vi "ProdaNG.TestValue.Set.vi"(8 "error in (no error)":errorcluster, 9 "ReleaseId":T1, 10 "TestValue":T2 {"minimum" format="%#.3f"; "maximum" format="%#.3f"}, 11 "dbHandleIn":i32) -> (0 "error out":errorcluster, 2 "TestValue out":T2 {"minimum" format="%#.3f"; "maximum" format="%#.3f"}, 3 "dbHandle":i32)   [LabVIEW 2016]
doc: "This function returns a product structure for a product, which is identified by a part and a serial number.\nImportant information: The field 'individual' was taken over from the field 'allgemein' of the legacy data directly. Because of this most products have the value 0 further on and only a few the value 1. \nParameter:\nhandle is an Integer, which is returned by the function Login() at the creation of a new connection.\nwabcoPartId is the Id of the part.\nserialNumber is the serial number of the product for the part above.\nproduct is a pointer on a product structure, which is filled if the returncode is 0. The structure must be defined in the calling program.\n\nReturncodes:\n0 No error\n< 0 ORACLE Error code\n6 (ERROR_INVALID_HANDLE) in case of an invalid handle\n1403 Record does not exist"
uses:
  Controls/ProdaNG.TestValue.ctl
  Controls/ProdaNG.ReleaseId.ctl
  Controls/ProdaNG.TestValueSize.ctl
  prodllNG.dll
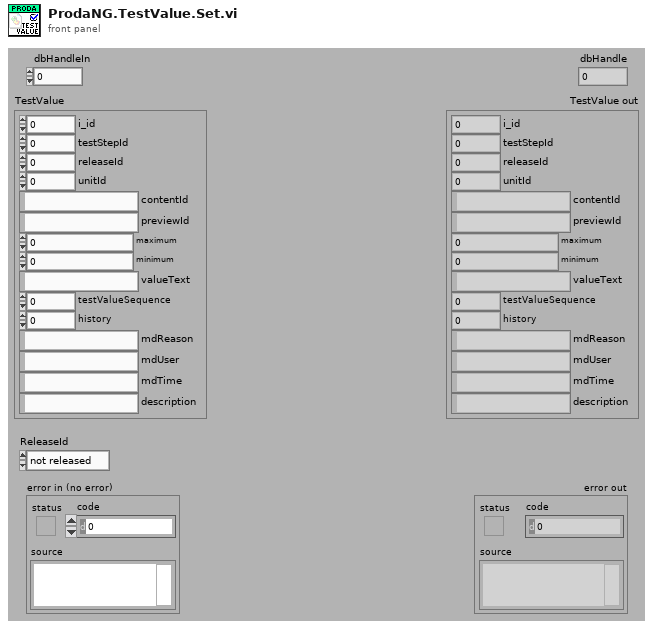
[diagram p1: front panel]
types:
  T1 = typedef "ProdaNG.ReleaseId.ctl" = enum16{"not released", "released", "was released"}
  T2 = typedef "ProdaNG.TestValue.ctl" = cluster{"i_id":i32, "testStepId":i32, "releaseId":i32, "unitId":i32, "contentId":string, "previewId":string, "maximum":dbl, "minimum":dbl, "valueText":string, "testValueSequence":i32, "history":i32, "mdReason":string, "mdUser":string, "mdTime":string, "description":string}
  T3 = typedef "ProdaNG.TestValueSize.ctl" = cluster{"i_id":i32, "testStepId":i32, "releaseId":i32, "unitId":i32, "contentId":i32, "previewId":i32, "maximum":i32, "minimum":i32, "valueText":i32, "testValueSequence":i32, "history":i32, "mdReason":i32, "mdUser":i32, "mdTime":i32, "description":i32}
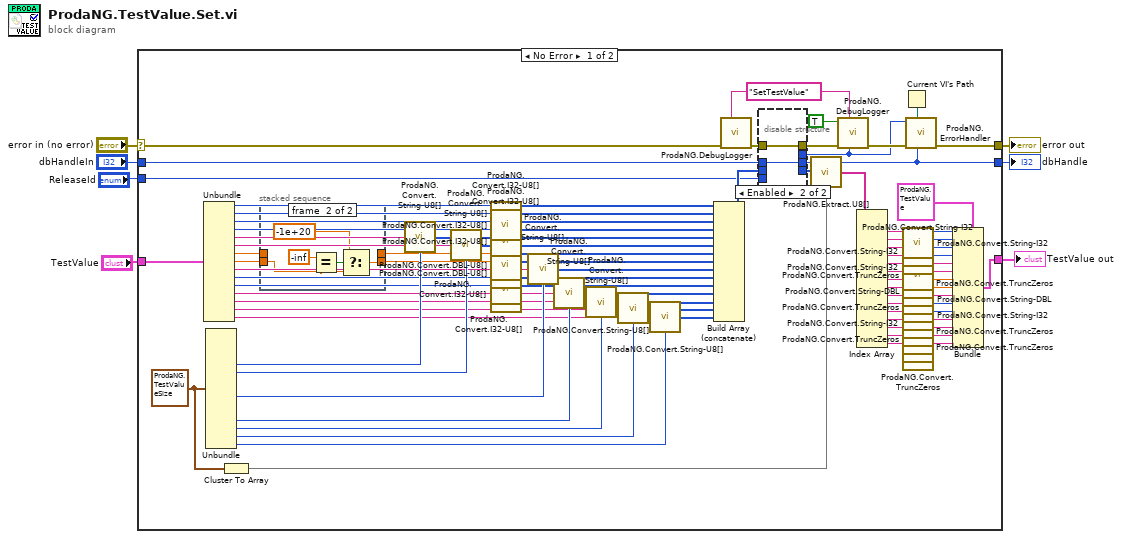
[diagram p0: block diagram]
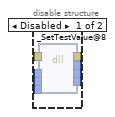
[diagram p2: hidden frame]
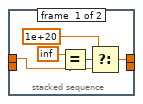
[diagram p3: hidden frame]
diagram:
  n1 = case shown="No Error" "error in (no error)" {
    selector: "error in (no error)" -> [w91 w118]
    tunnel: [w96 w118] -> w6
    tunnel: "dbHandleIn" -> [w93 w117]
    tunnel: [w94 w117] -> w4
    tunnel: "TestValue" -> [w60 _]
    tunnel: [w48 _] -> w3
    tunnel: "ReleaseId" -> [w12 _]
    frame No Error {
      w33 = T3 {"i_id"=4, "testStepId"=4, "releaseId"=4, "unitId"=4, "contentId"=16, "previewId"=16, "maximum"=8, "minimum"=8, "valueText"=258, "testValueSequence"=4, "history"=4, "mdReason"=514, "mdUser"=22, "mdTime"=24, "description"=514} ("TestStepValueSize")
      w87 = "SetTestValue" ("cmd")
      n2 = Unbundle(w60) -> ("i_id"=w83:i32, "testStepId"=w84:i32, "releaseId"=w56:i32, "unitId"=w55:i32, "contentId"=w81:string, "previewId"=w52:string, "maximum"=w11:dbl, "minimum"=w10:dbl, "valueText"=w31:string, "testValueSequence"=w28:i32, "history"=w27:i32, "mdReason"=w24:string, "mdUser"=w22:string, "mdTime"=w18:string, "description"=w17:string)
      n3 = Unbundle(w33) -> ("contentId"=w78:i32, "previewId"=w51:i32, "valueText"=w29:i32, "mdReason"=w23:i32, "mdUser"=w19:i32, "mdTime"=w15:i32, "description"=w16:i32)  [unwired: 8 out]
      n4 = Cluster To Array(cluster=w33) -> (array=w57:i32[])
      n5 = stacked-sequence {
        tunnel: w11 -> [w107 _]
        tunnel: w10 -> [_ w112]
        tunnel: [w109 _] -> w9
        tunnel: [_ w113] -> w8
        frame #0 {
          n6 = Equal?(x=inf, y=w107) -> (x = y?=w108:bool)
          n7 = Select(t=1e+20, s=w108, f=w107) -> (s? t:f=w109:dbl)
        }
        frame #1 {
          n8 = Equal?(x=-inf, y=w112) -> (x = y?=w114:bool)
          n9 = Select(t=-1e+20, s=w114, f=w112) -> (s? t:f=w113:dbl)
        }
      }
      n10 = call "ProdaNG.Convert.String-U8[].vi"("Input String"=w81, "Size"=w78) -> ("Output"=w80:u8[])
      n11 = call "ProdaNG.Convert.String-U8[].vi"("Input String"=w52, "Size"=w51) -> ("Output"=w49:u8[])
      n12 = call "ProdaNG.Convert.I32-U8[].vi"("32bit integer"=w83) -> ("unsigned byte array"=w82:u8[])  [unwired: 10 in]
      n13 = call "ProdaNG.Convert.I32-U8[].vi"("32bit integer"=w84) -> ("unsigned byte array"=w85:u8[])  [unwired: 10 in]
      n14 = call "ProdaNG.Convert.I32-U8[].vi"("32bit integer"=w56) -> ("unsigned byte array"=w53:u8[])  [unwired: 10 in]
      n15 = call "ProdaNG.Convert.I32-U8[].vi"("32bit integer"=w55) -> ("unsigned byte array"=w54:u8[])  [unwired: 10 in]
      n16 = call "ProdaNG.Convert.DBL-U8[].vi"("dbl"=w9) -> ("unsigned byte array"=w79:u8[])  [unwired: 10 in]
      n17 = call "ProdaNG.Convert.DBL-U8[].vi"("dbl"=w8) -> ("unsigned byte array"=w32:u8[])  [unwired: 10 in]
      n18 = call "ProdaNG.Convert.I32-U8[].vi"("32bit integer"=w28) -> ("unsigned byte array"=w26:u8[])  [unwired: 10 in]
      n19 = call "ProdaNG.Convert.I32-U8[].vi"("32bit integer"=w27) -> ("unsigned byte array"=w25:u8[])  [unwired: 10 in]
      n20 = call "ProdaNG.Convert.String-U8[].vi"("Input String"=w31, "Size"=w29) -> ("Output"=w30:u8[])
      n21 = call "ProdaNG.Convert.String-U8[].vi"("Input String"=w24, "Size"=w23) -> ("Output"=w20:u8[])
      n22 = call "ProdaNG.Convert.String-U8[].vi"("Input String"=w22, "Size"=w19) -> ("Output"=w21:u8[])
      n23 = call "ProdaNG.Convert.String-U8[].vi"("Input String"=w18, "Size"=w15) -> ("Output"=w14:u8[])
      n24 = call "ProdaNG.Convert.String-U8[].vi"("Input String"=w17, "Size"=w16) -> ("Output"=w13:u8[])
      n25 = Build Array (concatenate)(w82, w85, w53, w54, w80, w49, w79, w32, w30, w26, w25, w20, w21, w14, w13) -> (w59:u8[])
      n26 = call "ProdaNG.DebugLogger.vi"("cmd"=w87, "error in (no error)"=w91) -> ("error out"=w90:errorcluster)  [unwired: 9 in]
      n27 = disable-structure shown="Enabled" {
        disable-tunnel: [w104 w105] -> w94
        disable-tunnel: w93 -> [w103 w105]
        disable-tunnel: w90 -> [w102 w106]
        disable-tunnel: [w101 w106] -> w89
        disable-tunnel: [w100 _] -> w86
        disable-tunnel: w59 -> [w99 _]
        disable-tunnel: [w98 _] -> w58
        disable-tunnel: w12 -> [w97 _]
        frame Disabled {
          n28 = dll-call lib="D:/Maszup/WABCO/SVN/LaserMarkingStation/SOFTWARE/sources/Database/ProdaNG/prodllNG.dll" fn="_SetTestValue@8" ("ProDLL wrapper.dll:ProDLL_wrapper_GetWabcoParts_GetData")(error in=w102, "dbHandle"=w103, "testValuePtr"=w99, "releaseId"=w97) -> (error out=w101:errorcluster, "return type"=w100:i32, "dbHandle"=w104:i32, "testValuePtr"=w98:u8[])  [unwired: 3 in, 1 out]
        }
        frame Enabled {
        }
      }
      n29 = call "ProdaNG.Extract.U8[].vi"("unsigned byte array"=w58, "Sizes"=w57) -> ("Elements"=w77:string[])
      n30 = call "ProdaNG.DebugLogger.vi"("return type"=w86, "cmd"=w87, "error in (no error)"=w89, "done? (F)"=TRUE) -> ("error out"=w88:errorcluster)  [unwired: 7 in]
      n31 = Index Array(array=w77) -> (element #1=w76:string, element #2=w73:string, element #3=w72:string, element #4=w66:string, element #5=w63:string, element #6=w62:string, element #7=w67:string, element #8=w69:string, element #9=w46:string, element #10=w45:string, element #11=w44:string, element #12=w41:string, element #13=w39:string, element #14=w37:string, element #15=w36:string)  [unwired: 15 in]
      n32 = Current VI's Path() -> (path=w95:path)
      n33 = call "ProdaNG.Convert.String-I32.vi"("unsigned byte string"=w76) -> ("32bit integer"=w75:i32)  [unwired: 10 in]
      n34 = call "ProdaNG.Convert.String-I32.vi"("unsigned byte string"=w73) -> ("32bit integer"=w74:i32)  [unwired: 10 in]
      n35 = call "ProdaNG.Convert.String-I32.vi"("unsigned byte string"=w72) -> ("32bit integer"=w71:i32)  [unwired: 10 in]
      n36 = call "ProdaNG.Convert.String-I32.vi"("unsigned byte string"=w66) -> ("32bit integer"=w65:i32)  [unwired: 10 in]
      n37 = call "ProdaNG.Convert.TruncZeros.vi"("string with \\0s"=w63) -> ("LV string"=w64:string)  [unwired: 10 in]
      n38 = call "ProdaNG.Convert.TruncZeros.vi"("string with \\0s"=w62) -> ("LV string"=w61:string)  [unwired: 10 in]
      n39 = call "ProdaNG.Convert.String-DBL.vi"("unsigned byte string"=w67) -> ("dbl integer"=w68:dbl)  [unwired: 10 in]
      n40 = call "ProdaNG.Convert.String-DBL.vi"("unsigned byte string"=w69) -> ("dbl integer"=w70:dbl)  [unwired: 10 in]
      n41 = call "ProdaNG.Convert.TruncZeros.vi"("string with \\0s"=w46) -> ("LV string"=w47:string)  [unwired: 10 in]
      n42 = call "ProdaNG.Convert.String-I32.vi"("unsigned byte string"=w45) -> ("32bit integer"=w43:i32)  [unwired: 10 in]
      n43 = call "ProdaNG.Convert.String-I32.vi"("unsigned byte string"=w44) -> ("32bit integer"=w42:i32)  [unwired: 10 in]
      n44 = call "ProdaNG.Convert.TruncZeros.vi"("string with \\0s"=w41) -> ("LV string"=w40:string)  [unwired: 10 in]
      n45 = call "ProdaNG.Convert.TruncZeros.vi"("string with \\0s"=w39) -> ("LV string"=w38:string)  [unwired: 10 in]
      n46 = call "ProdaNG.Convert.TruncZeros.vi"("string with \\0s"=w37) -> ("LV string"=w35:string)  [unwired: 10 in]
      n47 = call "ProdaNG.Convert.TruncZeros.vi"("string with \\0s"=w36) -> ("LV string"=w34:string)  [unwired: 10 in]
      n48 = call "ProdaNG.ErrorHandler.vi"("dbHandleIn"=w94, "Path"=w95, "error in"=w88, "output_parameter"=w86) -> ("error out"=w96:errorcluster)  [unwired: 7 in]
      n49 = Bundle(cluster=T2 {"i_id"=0, "testStepId"=0, "releaseId"=0, "unitId"=0, "contentId"="", "previewId"="", "maximum"=0.0, "minimum"=0.0, "valueText"="", "testValueSequence"=0, "history"=0, "mdReason"="", "mdUser"="", "mdTime"="", "description"=""} ("TestStepValue"), "i_id"=w75, "testStepId"=w74, "releaseId"=w71, "unitId"=w65, "contentId"=w64, "previewId"=w61, "maximum"=w68, "minimum"=w70, "valueText"=w47, "testValueSequence"=w43, "history"=w42, "mdReason"=w40, "mdUser"=w38, "mdTime"=w35, "description"=w34) -> (w48:T2)
    }
    frame Error {
    }
  }
  "error out" <- w6
  "dbHandle" <- w4
  "TestValue out" <- w3
